vi "DO to Channel.vi"(10 "Output":T1) -> (2 "Channel":i32)   [LabVIEW 2020, in "HandsOnPi2040.lvlib"]
doc: "Converts the DigOut into the required channel."
uses:
  HandsOnPi2040.lvlib
  Public/DigOuts.ctl
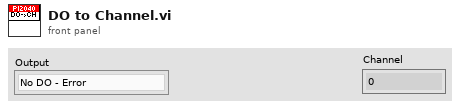
[diagram p1: front panel]
types:
  T1 = typedef "HandsOnPi2040.lvlib/DigOuts.ctl" = enum16{"No DO - Error", "DO1 (GPIO2)", "DO2 (GPIO3)", "DO3 (GPIO4)", "DO4 (GPIO5)", "BEEP (GPIO6)"}
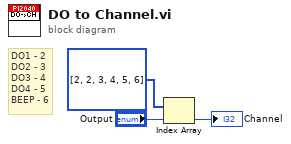
[diagram p0: block diagram]
diagram:
  # "DO1 - 2\nDO2 - 3\nDO3 - 4\nDO4 - 5\nBEEP - 6"
  n1 = Index Array(array=i32[] [2, 2, 3, 4, 5, 6], index="Output") -> (element=→"Channel":i32)
